vi "motor_block3.vi"(8 "error in":errorcluster, 10 "unit ID":u8, 11 "Modbus master in":refnum<class "Modbus Master.lvclass">) -> (0 "error out":errorcluster, 3 "Modbus master out":refnum<class "Modbus Master.lvclass">)   [LabVIEW 2020]
uses:
  <vilib>/NI/Modbus Library/API/Master/Modbus Master.lvclass
  C:/Program Files/National Instruments/LabVIEW 2020/vi.lib/NI/Modbus Library/API/Modbus API.lvclass
  <vilib>/NI/Modbus Library/API/Modbus API.lvclass/Modbus API.ctl
  <vilib>/NI/Modbus Library/Transmission Data Unit/Transmission Data Unit.lvclass/Transmission Data Unit.ctl
  <vilib>/NI/Modbus Library/Transmission Data Unit/Write Unit ID.vi
  <vilib>/NI/Modbus Library/API/Read Transmission Data Unit.vi
  <vilib>/NI/Modbus Library/API/Write Transmission Data Unit.vi
  status/emergency stop.vi
panel:
  out "current time":timestamp
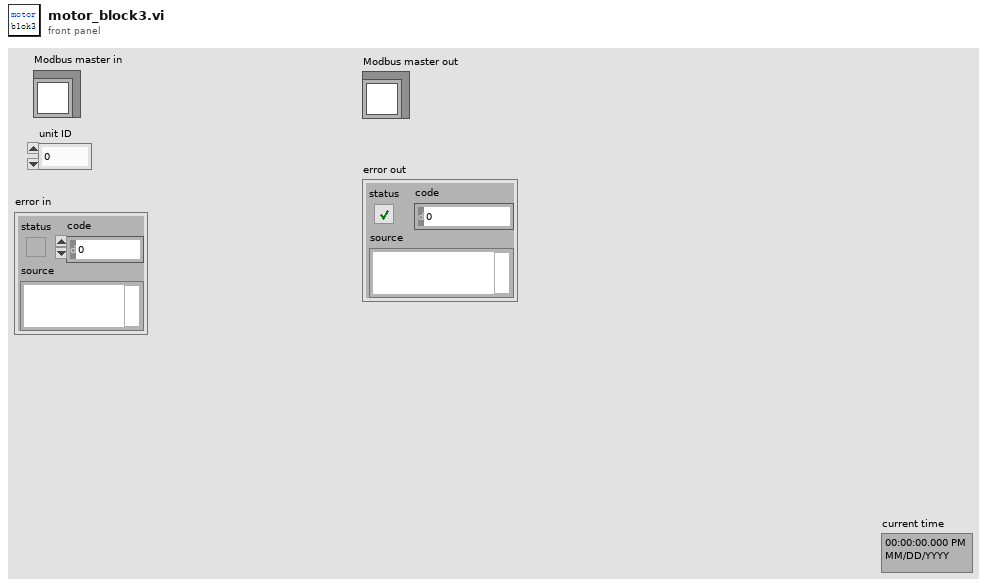
[diagram p1: front panel]
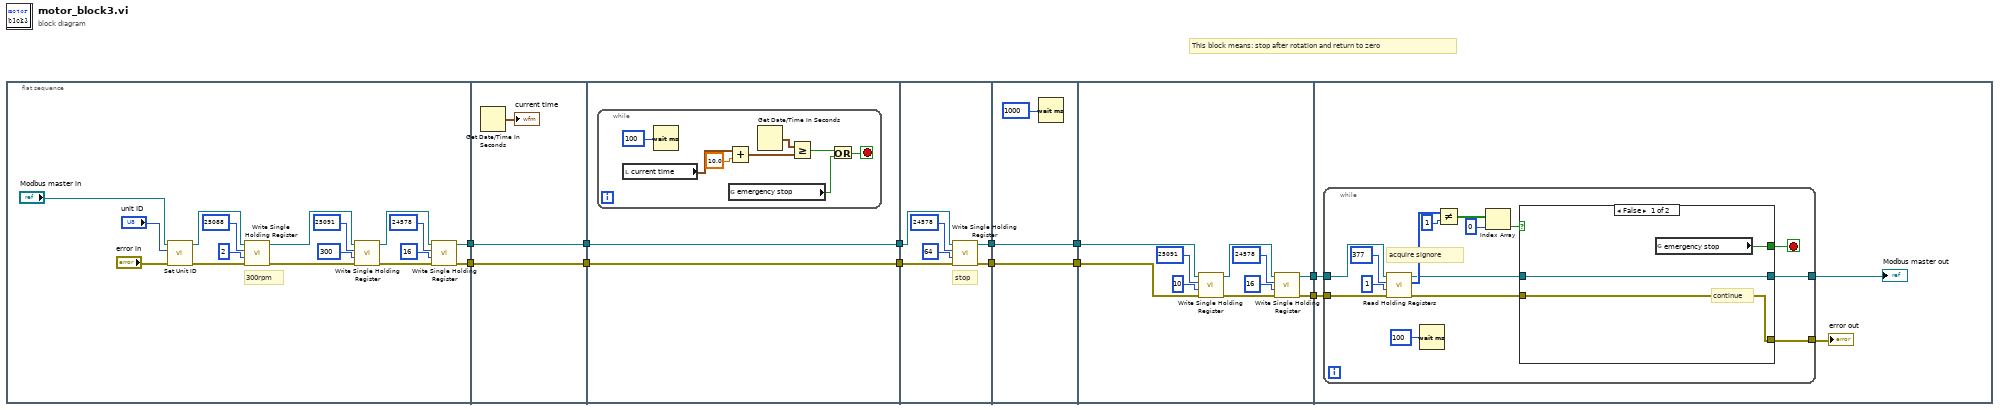
[diagram p0: block diagram]
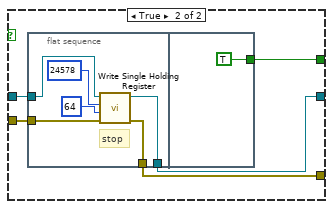
[diagram p2: hidden frame]
diagram:
  # "This block means: stop after rotation and return to zero"
  n1 = flat-sequence {
    tunnel: [w16] -> w4
    tunnel: [w15] -> w2
    tunnel: w4 -> [w32]
    tunnel: [w32] -> w3
    tunnel: w2 -> [w31]
    tunnel: [w31] -> w1
    tunnel: w3 -> [w34]
    tunnel: [w34] -> w12
    tunnel: [w33] -> w11
    tunnel: w1 -> [w33]
    tunnel: w12 -> [w46]
    tunnel: w11 -> [w45]
    tunnel: [w44] -> w8
    tunnel: [w43] -> w6
    tunnel: w8 -> [w51]
    tunnel: [w51] -> w7
    tunnel: w6 -> [w50]
    tunnel: [w50] -> w5
    tunnel: w7 -> [w55]
    tunnel: w5 -> [w54]
    tunnel: [w53] -> w10
    tunnel: [w52] -> w9
    tunnel: w10 -> [w65]
    tunnel: w9 -> [w64]
    frame #0 {
      # "300rpm"
      n2 = call <vilib>:"Set Unit ID.vi"("error in"="error in", "unit ID"="unit ID", "Modbus master in"="Modbus master in") -> ("error out"=w28:errorcluster, "Modbus master out"=w27:refnum<class "Modbus Master.lvclass">)  [unwired: 7 in]
      n3 = call-dynamic "Write Single Holding Register.vi"("error in"=w28, "register to write"=u16 2 ("address"), "address"=u16 25088, "Modbus master in"=w27) -> ("error out"=w26:errorcluster, "Modbus master out"=w25:refnum<class "Modbus Master.lvclass">)  [unwired: 6 in]
      n4 = call-dynamic "Write Single Holding Register.vi"("error in"=w26, "register to write"=u16 300 ("address"), "address"=u16 25091, "Modbus master in"=w25) -> ("error out"=w17:errorcluster, "Modbus master out"=w18:refnum<class "Modbus Master.lvclass">)  [unwired: 6 in]
      n5 = call-dynamic "Write Single Holding Register.vi"("error in"=w17, "register to write"=u16 16 ("address"), "address"=u16 24578, "Modbus master in"=w18) -> ("error out"=w15:errorcluster, "Modbus master out"=w16:refnum<class "Modbus Master.lvclass">)  [unwired: 6 in]
    }
    frame #1 {
      n6 = Get Date/Time In Seconds() -> (seconds since 1Jan1904=→"current time":timestamp)
    }
    frame #2 {
      n7 = while {
        stop <- w35 stop-if-true
        n8 = local read "current time"() -> (w41:timestamp)
        n9 = Wait (ms)(milliseconds to wait=u32 100 ("millisecond timer value")) -> ()  [unwired: 1 out]
        n10 = Add(x=w41, y=10.0) -> (x+y=w39:timestamp)
        n11 = global read "emergency stop.vi" "emergency stop"() -> (w36:bool)
        n12 = Get Date/Time In Seconds() -> (seconds since 1Jan1904=w38:timestamp)
        n13 = Greater Or Equal?(x=w38, y=w39) -> (x >= y?=w37:bool)
        n14 = Or(x=w37, y=w36) -> (x .or. y?=w35:bool)
      }
    }
    frame #3 {
      # "stop"
      n15 = call-dynamic "Write Single Holding Register.vi"("error in"=w45, "register to write"=u16 64 ("address"), "address"=u16 24578, "Modbus master in"=w46) -> ("error out"=w43:errorcluster, "Modbus master out"=w44:refnum<class "Modbus Master.lvclass">)  [unwired: 6 in]
    }
    frame #4 {
      n16 = Wait (ms)(milliseconds to wait=u32 1000) -> ()  [unwired: 1 out]
    }
    frame #5 {
      n17 = call-dynamic "Write Single Holding Register.vi"("error in"=w54, "register to write"=u16 10 ("address"), "address"=u16 25091, "Modbus master in"=w55) -> ("error out"=w56:errorcluster, "Modbus master out"=w57:refnum<class "Modbus Master.lvclass">)  [unwired: 6 in]
      n18 = call-dynamic "Write Single Holding Register.vi"("error in"=w56, "register to write"=u16 16 ("address"), "address"=u16 24578, "Modbus master in"=w57) -> ("error out"=w52:errorcluster, "Modbus master out"=w53:refnum<class "Modbus Master.lvclass">)  [unwired: 6 in]
    }
    frame #6 {
      n19 = while {
        tunnel: [w71] -> w63
        tunnel: [w70] -> w62
        tunnel: w65 -> [w69]
        tunnel: w64 -> [w68]
        stop <- w72 stop-if-true
        # "acquire signore"
        n20 = call-dynamic "Read Holding Registers.vi"("error in"=w68, "number of inputs"=u16 1 ("address"), "starting address"=u16 377 ("address"), "Modbus master in"=w69) -> ("error out"=w73:errorcluster, "register values"=w79:u16[], "Modbus master out"=w74:refnum<class "Modbus Master.lvclass">)  [unwired: 5 in]
        n21 = Wait (ms)(milliseconds to wait=u32 100) -> ()  [unwired: 1 out]
        n22 = Not Equal?(x=w79, y=u16 1 ("number of inputs")) -> (x != y?=w77:bool[])
        n23 = Index Array(array=w77, index=0) -> (element=w75:bool)
        n24 = case shown="False" w75 {
          tunnel: w74 -> [w83 w88]
          tunnel: w73 -> [w82 w87]
          tunnel: [w81 w86] -> w72
          tunnel: [w83 w85] -> w71
          tunnel: [w82 w84] -> w70
          frame False {
            # "continue"
            n25 = global read "emergency stop.vi" "emergency stop"() -> (w81:bool)
          }
          frame True {
            n26 = flat-sequence {
              tunnel: w88 -> [w92]
              tunnel: w87 -> [w91]
              tunnel: [w90] -> w85
              tunnel: [w89] -> w84
              tunnel: [TRUE] -> w86
              frame #0 {
                # "stop"
                n27 = call-dynamic "Write Single Holding Register.vi"("error in"=w91, "register to write"=u16 64 ("address"), "address"=u16 24578, "Modbus master in"=w92) -> ("error out"=w89:errorcluster, "Modbus master out"=w90:refnum<class "Modbus Master.lvclass">)  [unwired: 6 in]
              }
              frame #1 {
              }
            }
          }
        }
      }
      "Modbus master out" <- w63
      "error out" <- w62
    }
  }
